vi "Determine good page.vi"(10 "Page":i32[](array[numeric]), 11 "Rules":i32[][](array[numeric])) -> (3 "Correct Order Out":bool)   [LabVIEW 2024]
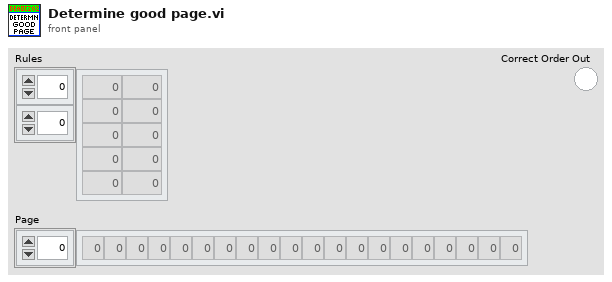
[diagram p1: front panel]
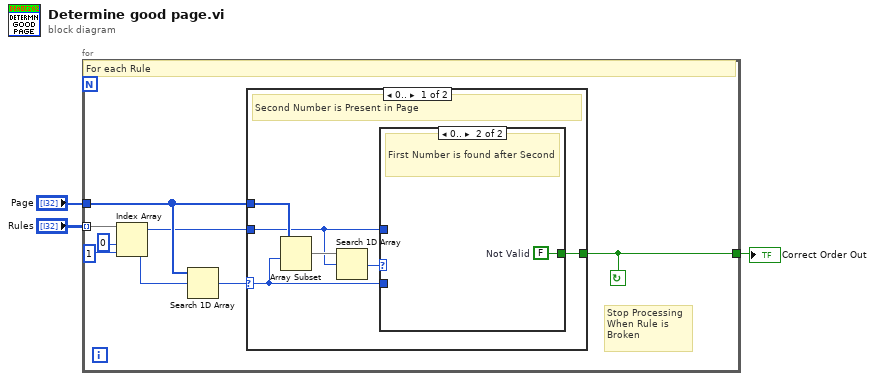
[diagram p0: block diagram]
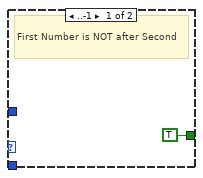
[diagram p2: hidden frame]
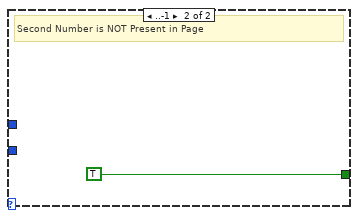
[diagram p3: hidden frame]
diagram:
  n1 = for {
    tunnel: "Rules" -> [w11] mode=indexing
    tunnel: [w4] -> w1
    tunnel: "Page" -> [w6]
    stop <- w4 continue-if-true
    # "Stop Processing\nWhen Rule is \nBroken"
    # "For each Rule"
    n2 = Index Array(array=w11, index #1=0 ("index"), index #2=1 ("index")) -> (element #1=w5:i32, element #2=w8:i32)
    n3 = Search 1D Array(1D array=w6, element=w8) -> (index of element=w7:i32)  [unwired: 1 in]
    n4 = case shown="0.." w7 {
      selector: w7 -> [w15 _]
      tunnel: w6 -> [w14 _]
      tunnel: w5 -> [w12 _]
      tunnel: [w13 TRUE ("Not Valid")] -> w4
      frame 0.. {
        # "Second Number is Present in Page"
        n5 = Array Subset(array=w14, index=w15) -> (w17:i32[])  [unwired: 1 in]
        n6 = Search 1D Array(1D array=w17, element=w12) -> (index of element=w16:i32)  [unwired: 1 in]
        n7 = case shown="0.." w16 {
          tunnel: w15 -> [_ _]
          tunnel: [TRUE ("Not Valid") w19] -> w13
          tunnel: w12 -> [_ _]
          frame ..-1 {
            # "First Number is NOT after Second"
          }
          frame 0.. {
            w19 = FALSE  # Not Valid
            # "First Number is found after Second"
          }
        }
      }
      frame ..-1 {
        # "Second Number is NOT Present in Page"
      }
    }
  }
  "Correct Order Out" <- w1
